vi "op_rel_v4.vi"() -> ()   [LabVIEW 2009]
panel:
  in  "Slide":u8(slide)=8 scale=0.0..9.0
  out "L":bool=TRUE
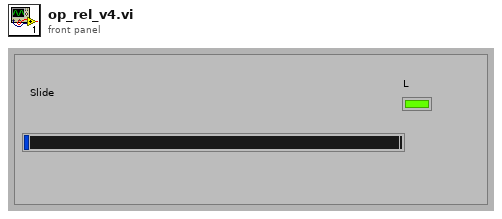
[diagram p1: front panel]
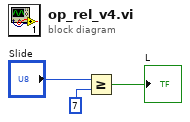
[diagram p0: block diagram]
diagram:
  n1 = Greater Or Equal?(x="Slide", y=7) -> (x >= y?=→"L":bool)
